vi "PH_GetPowermeterInformation.get and prepare Info.vi"(5 "error in":errorcluster) -> (15 "ColHdrs[]":string[](array[string])=["Sixpack Instance", "Axis"], 16 "RowHdrs[]":string[](array[string]), 17 "ItemNames":string[][](array[string]), 18 "Row Cell BG":u32[](array[numeric]), 19 "error out":errorcluster)   [LabVIEW 2014, in "PH_GetPowermeterInformation.lvlib"]
doc: "This VI is reading out information from the database and prepares it for the visualisation on the GUI."
uses:
  PH_GetPowermeterInformation.lvlib
  PH_Basics/PH_Common/PH_Common.lvlib
  CS_Core/CSSystem/CSSystemLib/CSSystemLib.lvlib
  PH_Basics/PH_Powermeter_BaseClass/PH_Powermeter_BaseClass.lvlib
  PH_Devices/PH_gentec_M-Link/PH_gentec_M-Link.lvlib
  PH_Devices/PH_gentec_Powermeter/PH_gentec_Powermeter.lvlib
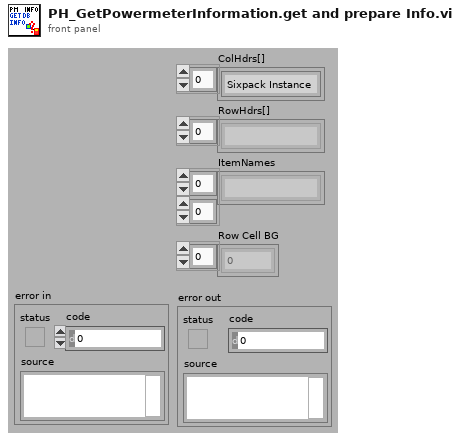
[diagram p1: front panel]
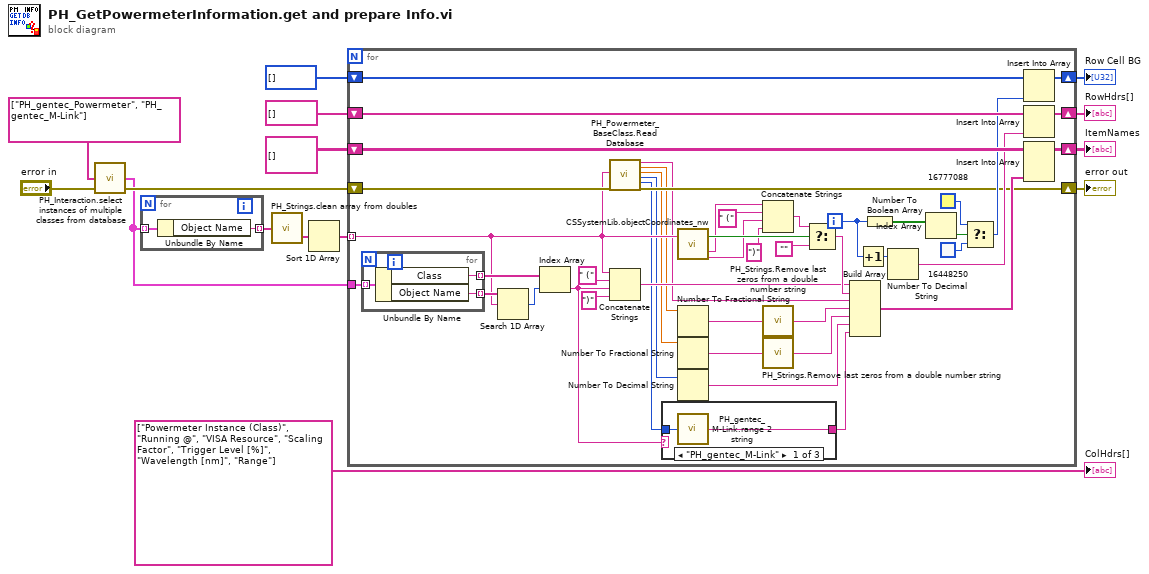
[diagram p0: block diagram]
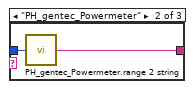
[diagram p2: hidden frame]
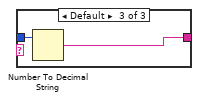
[diagram p3: hidden frame]
diagram:
  n1 = call "PH_Interaction.select instances of multiple classes from database.vi"("error in (no error)"="error in", "Classes Input"=string[] ["PH_gentec_Powermeter", "PH_gentec_M-Link"]) -> ("error out"=w7:errorcluster, "Query Result"=w1:cluster{"Object Name":string, "Class":string}[])  [unwired: 2 in]
  n2 = for {
    tunnel: w1 -> [w17] mode=indexing
    tunnel: [w16] -> w6 mode=indexing
    n3 = Unbundle By Name(w17) -> ("Object Name"=w16:string)
  }
  n4 = call "PH_Strings.clean array from doubles.vi"("Array Input"=w6) -> ("Cleaned Array Output"=w5:string[])  [unwired: 1 out]
  n5 = Sort 1D Array(array=w5) -> (sorted array=w4:string[])
  n6 = for {
    tunnel: w4 -> [w30] mode=indexing
    shift-right: [w62] -> w11
    shift-left: string[][] [] -> [w61]
    shift-right: [w58] -> w13
    shift-left: string[] [] -> [w59]
    shift-right: [w56] -> w15
    shift-left: u32[] [] -> [w55]
    shift-right: [w31] -> w2
    shift-left: w7 -> [w32]
    tunnel: w1 -> [w39]
    i -> [w45]
    n7 = for {
      tunnel: w39 -> [w71] mode=indexing
      tunnel: [w70] -> w38 mode=indexing
      tunnel: [w69] -> w37 mode=indexing
      n8 = Unbundle By Name(w71) -> ("Class"=w69:string, "Object Name"=w70:string)
    }
    n9 = Search 1D Array(1D array=w38, element=w30) -> (index of element=w36:i32)  [unwired: 1 in]
    n10 = Index Array(array=w37, index=w36) -> (element=w20:string)
    n11 = call "PH_Powermeter_BaseClass.Read Database.vi"("Instance Name"=w30, "error in"=w32) -> ("VISA Resource"=w29:string, "Scaling Factor"=w28:dbl, "Trigger Level [%]"=w26:dbl, "Wavelength [nm]"=w24:u32, "Range"=w22:u32, "error out"=w31:errorcluster)  [unwired: 12 in]
    n12 = Concatenate Strings(w30, " (" ("string"), w20, ")" ("string")) -> (w33:string)
    n13 = case shown="\"PH_gentec_M-Link\"" w20 {
      tunnel: w22 -> [w64 w66 w68]
      tunnel: [w63 w65 w67] -> w21
      frame "PH_gentec_M-Link" {
        n14 = call "PH_gentec_M-Link.range 2 string.vi"("Range"=w64) -> ("Range as string"=w63:string)
      }
      frame "PH_gentec_Powermeter" {
        n15 = call "PH_gentec_Powermeter.range 2 string.vi"("Range"=w66) -> ("Range as string"=w65:string)
      }
      frame Default {
        n16 = Number To Decimal String(number=w68) -> (decimal integer string=w67:string)  [unwired: 1 in]
      }
    }
    n17 = call "CSSystemLib.objectCoordinates_nw.vi"("name"=w30) -> ("obj exists"=w54:bool, "systemID"=w51:string, "node"=w48:string)  [unwired: 15 in, 1 out]
    n18 = Number To Fractional String(number=w28) -> (F-format string=w27:string)  [unwired: 3 in]
    n19 = Number To Fractional String(number=w26) -> (F-format string=w25:string)  [unwired: 3 in]
    n20 = Number To Decimal String(number=w24) -> (decimal integer string=w23:string)  [unwired: 1 in]
    n21 = Concatenate Strings(w51, " (" ("string"), w48, ")" ("string")) -> (w50:string)
    n22 = call "PH_Strings.Remove last zeros from a double number string.vi"("String in"=w27) -> ("String out"=w19:string)
    n23 = call "PH_Strings.Remove last zeros from a double number string.vi"("String in"=w25) -> ("String out"=w18:string)
    n24 = Select(t=w50, s=w54, f="") -> (s? t:f=w52:string)
    n25 = Build Array(w33, w52, w29, w19, w18, w23, w21) -> (w46:string[])
    n26 = Increment(x=w45) -> (x+1=w44:i32)
    n27 = Number To Boolean Array(number=w45) -> (Boolean array=w42:bool[])
    n28 = Number To Decimal String(number=w44) -> (decimal integer string=w60:string)  [unwired: 1 in]
    n29 = Index Array(array=w42) -> (element=w43:bool)  [unwired: 1 in]
    n30 = Select(t=u32 16777088 ("Color Box"), s=w43, f=u32 16448250 ("Color Box")) -> (s? t:f=w57:u32)
    n31 = Insert Into Array(array=w55, new element=w57) -> (w56:u32[])  [unwired: 1 in]
    n32 = Insert Into Array(array=w59, new element=w60) -> (w58:string[])  [unwired: 1 in]
    n33 = Insert Into Array(array=w61, new element=w46) -> (w62:string[][])  [unwired: 2 in]
  }
  "error out" <- w2
  "Row Cell BG" <- w15
  "RowHdrs[]" <- w13
  "ItemNames" <- w11
  "ColHdrs[]" <- string[] ["Powermeter Instance (Class)", "Running @", "VISA Resource", "Scaling Factor", "Trigger Level [%]", "Wavelength [nm]", "Range"] ("new element/subarray")
